vi "Add Classes.vi"(8 "error in (no error)":errorcluster, 10 "Classes":string[](array[string]), 11 "Nav Route in":refnum<class "Nav Route.lvclass">) -> (0 "error out":errorcluster, 3 "Nav Route out":refnum<class "Nav Route.lvclass">)   [LabVIEW 2020, in "Volatus.lvlib" / "Nav Route.lvclass"]
uses:
  Nav Route.lvclass
  Nav Route.lvclass/Nav Route.ctl
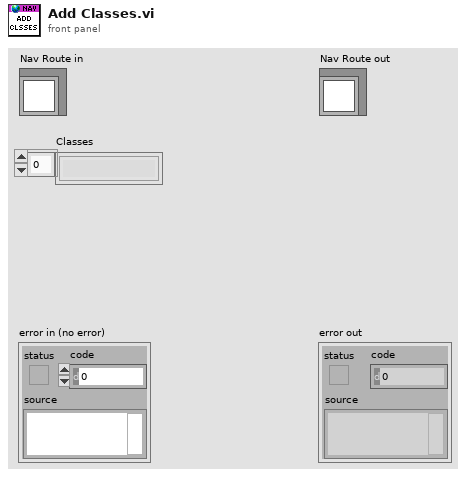
[diagram p1: front panel]
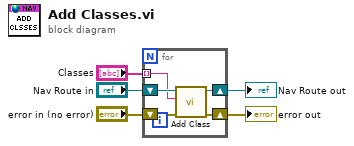
[diagram p0: block diagram]
diagram:
  n1 = for {
    shift-right: [w7] -> w2
    shift-left: "Nav Route in" -> [w10]
    shift-right: [w8] -> w3
    shift-left: "error in (no error)" -> [w9]
    tunnel: "Classes" -> [w6] mode=indexing
    n2 = call "Add Class.vi"("error in (no error)"=w9, "Class"=w6, "Nav Route in"=w10) -> ("error out"=w8:errorcluster, "Nav Route out"=w7:refnum<class "Nav Route.lvclass">)  [unwired: 7 in]
  }
  "error out" <- w3
  "Nav Route out" <- w2
